vi "errorDisplay.vi"(9 "error path index in":i32, 10 "error?":bool, 11 "string check in":string) -> (1 "string check":string, 2 "path index":string, 3 "errorInString?":bool)   [LabVIEW 2015]
panel:
  out "error out":errorcluster
  in  "error in (no error)":errorcluster
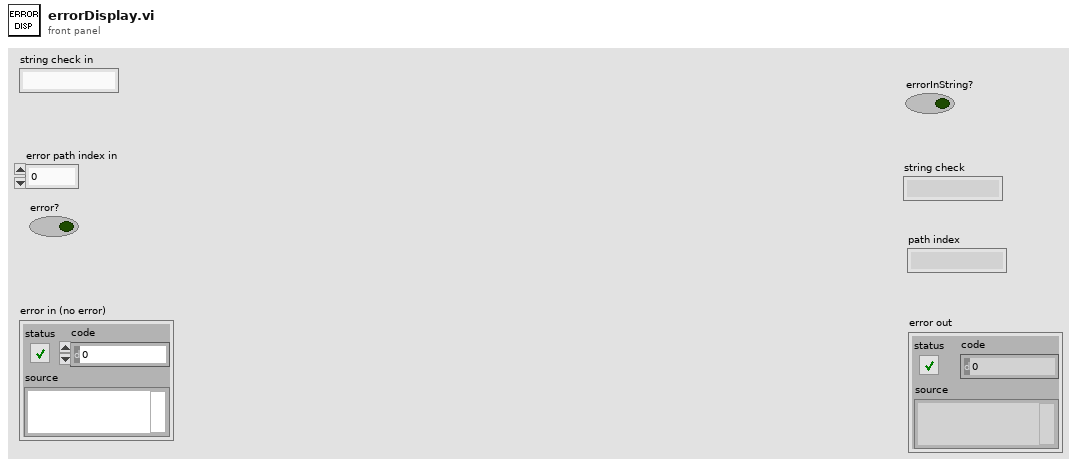
[diagram p1: front panel]
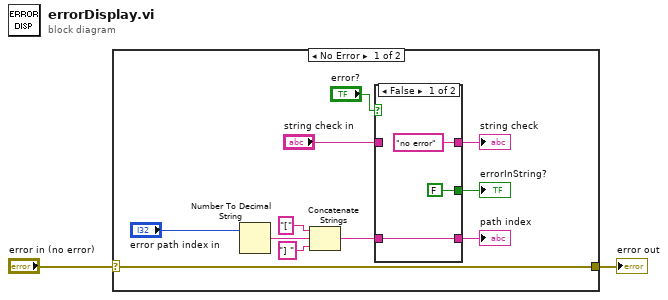
[diagram p0: block diagram]
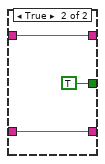
[diagram p2: hidden frame]
diagram:
  n1 = case shown="No Error" "error in (no error)" {
    selector: "error in (no error)" -> [w8 w20]
    tunnel: [w8 w20] -> w1
    frame No Error {
      n2 = Number To Decimal String(number="error path index in") -> (decimal integer string=w7:string)  [unwired: 1 in]
      n3 = Concatenate Strings("[" ("string"), w7, "] " ("string")) -> (w3:string)
      n4 = case shown="False" "error?" {
        tunnel: w3 -> [w15 w19]
        tunnel: [FALSE ("true") TRUE ("true")] -> w11
        tunnel: "string check in" -> [_ w18]
        tunnel: ["no error" ("string check in") w18] -> w9
        tunnel: [w15 w19] -> w10
        frame False {
        }
        frame True {
        }
      }
      "errorInString?" <- w11
      "path index" <- w10
      "string check" <- w9
    }
    frame Error {
    }
  }
  "error out" <- w1
